vi "ToTrace.vi"(0 "ToTrace":string, 1 "TraceRef":refnum<vi>, 11 "error in (no error)":errorcluster) -> (15 "error out":errorcluster)   [LabVIEW 2017]
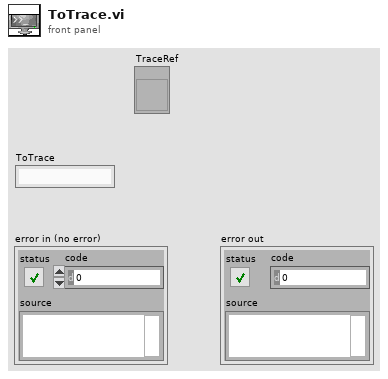
[diagram p1: front panel]
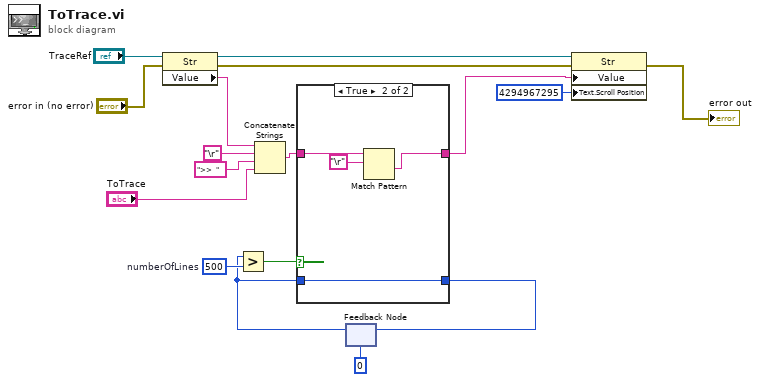
[diagram p0: block diagram]
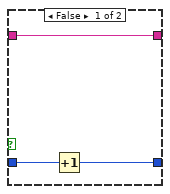
[diagram p2: hidden frame]
diagram:
  w11 = 500  # numberOfLines
  n1 = property class="Str"(reference="TraceRef", error in="error in (no error)") -> (reference out=w15:refnum<vi>, error out=w14:errorcluster, "Value"=w5:string)
  n2 = Concatenate Strings(w5, "\r", ">>  " ("string"), "ToTrace") -> (w4:string)
  n3 = feedback #1(0) -> (w9:i32)
  n4 = Greater?(x=w9, y=w11) -> (0:w10:bool)
  n5 = case shown="True" w10 {
    tunnel: w9 -> [w20 w24]
    tunnel: [w19 w24] -> w8
    tunnel: w4 -> [w18 w22]
    tunnel: [w18 w21] -> w3
    frame False {
      n6 = Increment(x=w20) -> (x+1=w19:i32)
    }
    frame True {
      n7 = Match Pattern(string=w22, regular expression="\r") -> (after substring=w21:string)  [unwired: 1 in, 3 out]
    }
  }
  n8 = feedback-in #1(w8) -> ()
  n9 = property class="Str"(reference=w15, error in=w14, "Value"=w3, "Text.Scroll Position"=u32 4294967295) -> (error out=→"error out":errorcluster)  [unwired: 1 out]
